vi "Ramp Up or Down.vi"(0 "Array":dbl[](array[numeric]), 2 "Down at end":bool, 7 "Sampling rate (Hz)":dbl, 9 "Ramp (ms)":dbl=5.0, 11 "Ramp up?":bool=TRUE, 12 "Start (0)":dbl, 13 "End (1)":dbl=1.0) -> (4 "Ramped array":dbl[](array[numeric]), 8 "Ramp length":u32)   [LabVIEW 2020]
uses:
  <vilib>/Analysis/NI_AALBase.lvlib
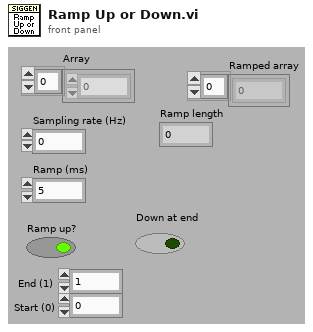
[diagram p1: front panel]
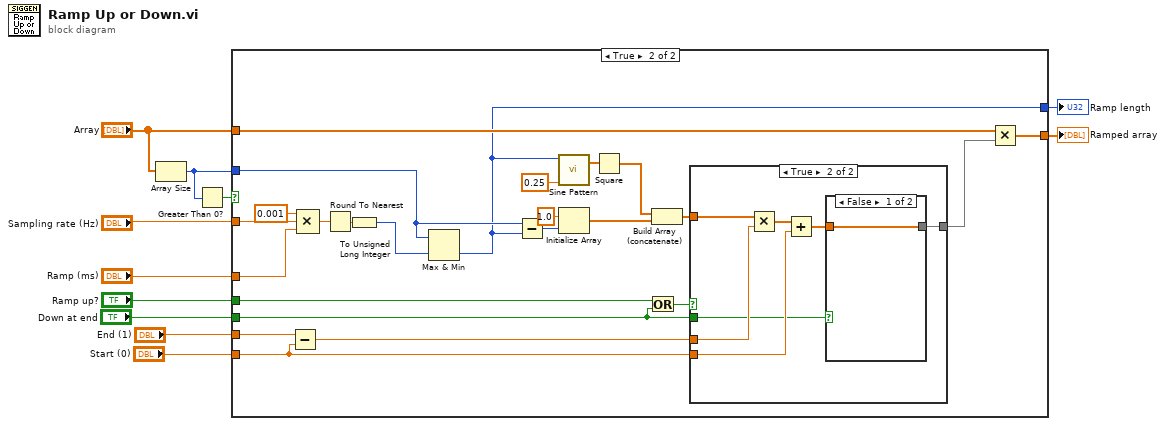
[diagram p0: block diagram]
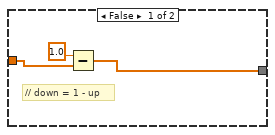
[diagram p3: hidden frame]
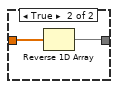
[diagram p4: hidden frame]
diagram:
  n1 = Array Size(array="Array") -> (size(s)=w7:i32)
  n2 = Greater Than 0?(x=w7) -> (x > 0?=w8:bool)
  n3 = case shown="True" w8 {
    tunnel: "Ramp up?" -> [_ w15]
    tunnel: "Sampling rate (Hz)" -> [_ w30]
    tunnel: "Ramp (ms)" -> [_ w27]
    tunnel: w7 -> [_ w24]
    tunnel: "Array" -> [w12 w22]
    tunnel: [w12 w20] -> w5
    tunnel: "Start (0)" -> [_ w18]
    tunnel: "End (1)" -> [_ w19]
    tunnel: "Down at end" -> [_ w14]
    tunnel: [_ w13] -> w1
    frame False {
    }
    frame True {
      n4 = Subtract(x=w19, y=w18) -> (x-y=w17:dbl)
      n5 = Compound Arithmetic op=MULTIPLY(0.001 ("value"), w30, w27) -> (w31:dbl)
      n6 = Round To Nearest(number=w31) -> (nearest integer value=w36:dbl)
      n7 = To Unsigned Long Integer(number=w36) -> (unsigned 32bit integer=w23:u32)
      n8 = Max & Min(x=w24, y=w23) -> (min(x,y)=w13:u32)  [unwired: 1 out]
      n9 = Subtract(x=w24, y=w13) -> (x-y=w35:u32)
      n10 = call <vilib>:"Sine Pattern.vi"("cycles"=0.25, "samples"=w13) -> ("Sinusoidal Pattern"=w26:dbl[])  [unwired: 2 in, 1 out]
      n11 = Initialize Array(1.0 ("element"), w35) -> (w33:dbl[])
      n12 = Square(x=w26) -> (x^2=w25:dbl[])
      n13 = Or(x=w15, y=w14) -> (x .or. y?=w16:bool)
      n14 = Build Array (concatenate)(w25, w33) -> (w32:dbl[])
      n15 = case shown="True" w16 {
        tunnel: w32 -> [w38 w46]
        tunnel: [w37 w41] -> w21
        tunnel: w18 -> [_ w45]
        tunnel: w17 -> [_ w43]
        tunnel: w14 -> [_ w40]
        frame False {
          # "// down = 1 - up"
          n16 = Subtract(x=1.0, y=w38) -> (x-y=w37:dbl[])
        }
        frame True {
          n17 = Multiply(x=w46, y=w43) -> (x*y=w44:dbl[])
          n18 = Add(x=w44, y=w45) -> (x+y=w42:dbl[])
          n19 = case shown="False" w40 {
            tunnel: w42 -> [w47 w49]
            tunnel: [w47 w48] -> w41
            frame False {
            }
            frame True {
              n20 = Reverse 1D Array(array=w49) -> (reversed array=w48:dbl[])
            }
          }
        }
      }
      n21 = Multiply(x=w22, y=w21) -> (x*y=w20:dbl[])
    }
  }
  "Ramped array" <- w5
  "Ramp length" <- w1
